vi "Launch Chart.vi"   [LabVIEW 2017]
uses:
  ExampleSimpleRootModel/SimpleRootModel.lvclass
  C:/Git/mva-framework/gpm_packages/@cs/mva-core/Source/IObserver/IObserver/IObserver.lvclass
  C:/Git/mva-framework/gpm_packages/@cs/mva-core/Source/IModel/IModel/IModel.lvclass
  SimpleChart/SimpleChart.lvclass
  C:/Git/mva-framework/gpm_packages/@cs/mva-viewable/Source/IViewable/IViewable/IViewable.lvclass
  gpm_packages/@cs/mva-viewable/Source/IViewModel/IViewModel/IViewModel.lvclass
  C:/Git/mva-framework/gpm_packages/@cs/mva-viewable/Source/IViewManager/IViewManager/IViewManager.lvclass
  C:/Program Files (x86)/National Instruments/LabVIEW 2017/vi.lib/ActorFramework/Actor/Actor.lvclass
  gpm_packages/@cs/mva-core/Source/Mediator/Mediator/Mediator.lvclass
  C:/Git/mva-framework/gpm_packages/@cs/mva-core/Source/IMediator/IMediator/IMediator.lvclass
  <vilib>/ActorFramework/Message Enqueuer/Message Priority.ctl
  gpm_packages/@cs/mva-viewable/Source/IViewable/IViewable/View Position Enum.ctl
  ExampleSimpleRootModel/SimpleRootModel.lvclass/SimpleRootModel.ctl
  gpm_packages/@cs/event-logger/Source/Composed Log/LoggerReference/LoggerReference.lvclass/LoggerReference.ctl
  gpm_packages/@cs/mva-core/Source/IObserver/IObserver/IObserver.lvclass/IObserver.ctl
  gpm_packages/@cs/mva-core/Source/IMediator/IMediator/IMediator.lvclass/IMediator.ctl
  gpm_packages/@cs/mva-viewable/Source/IViewModel/IViewModel/IViewModel.lvclass/IViewModel.ctl
  gpm_packages/@cs/mva-viewable/Source/IViewManager/IViewManager Messages/Launch Nested Views Msg/Launch Nested Views Msg.lvclass/Launch Nested Views Msg.ctl
  gpm_packages/@cs/mva-viewable/Source/IViewManager/IViewManager/IViewManager.lvclass/IViewManager.ctl
  gpm_packages/@cs/mva-viewable/Source/IViewable/IViewable Messages/Open Front Panel Msg/Open Front Panel Msg.lvclass/Open Front Panel Msg.ctl
  <vilib>/ActorFramework/Message Enqueuer/Message Enqueuer.lvclass/Message Enqueuer.ctl
  158084ce-0d1a-4c6f-81cb-d0b1039f64dd.vi
  158084ce-0d1a-4c6f-81cb-d0b1039f64dd.vi/7a735fd6-0766-4914-b472-33d23f5eb4e6.vi
  gpm_packages/@cs/mva-core/Source/IObserver/IObserver/Configure Observer Logging.vi
  gpm_packages/@cs/mva-viewable/Source/IViewModel/IViewModel/Write Startup Model-View Configuration.vi
  gpm_packages/@cs/mva-core/Source/IMediator/IMediator/Configure Mediator.vi
  <vilib>/ActorFramework/Message Enqueuer/Enqueue.vi
  gpm_packages/@cs/event-logger/Source/Composed Log/LoggerReference/Return Aggregate Queues.vi
  gpm_packages/@cs/event-logger/Source/Composed Log/LoggerReference/Add Aggregate Log.vi
  158084ce-0d1a-4c6f-81cb-d0b1039f64dd.vi/7a735fd6-0766-4914-b472-33d23f5eb4e6.vi/481b5bb9-d2a3-4a79-b1b5-84a351928f52.vi
  gpm_packages/@cs/mva-viewable/Source/IViewManager/IViewManager Messages/Launch Nested Views Msg/Pack Launch Nested Views Msg.vi
  gpm_packages/@cs/mva-viewable/Source/IViewManager/IViewManager/Write Startup Launch Nested Views Msg.vi
  gpm_packages/@cs/event-logger/Source/Composed Log/LoggerReference/Send Add Sink.vi
  gpm_packages/@cs/event-logger/Source/Text File Sink/Text File Sink.lvclass
  C:/Git/mva-framework/gpm_packages/@cs/event-logger/Source/Composed Log/Log Sink/Log Sink.lvclass
  gpm_packages/@cs/mva-viewable/Source/IViewable/IViewable Messages/Open Front Panel Msg/Open Front Panel Msg.lvclass
  C:/Program Files (x86)/National Instruments/LabVIEW 2017/vi.lib/ActorFramework/Message/Message.lvclass
  gpm_packages/@cs/event-logger/Source/Composed Log/Application Logger/Launch Worker Loop.vi
  gpm_packages/@cs/event-logger/Source/Composed Log/LoggerReference/Initialize Logger Instance.vi
  <vilib>/ActorFramework/Message Priority Queue/Priority Enqueue.vi
  gpm_packages/@cs/event-logger/Source/Composed Log/LoggerReference/LoggerReference.lvclass
  gpm_packages/@cs/event-logger/Source/Composed Log/IErrorFormat/IErrorFormat.lvclass
  gpm_packages/@cs/event-logger/Source/Composed Log/Log Sink/Log Sink.lvclass
  gpm_packages/@cs/mva-viewable/Source/IViewable/IApplicationStyle/IApplicationStyle.lvclass
  gpm_packages/@cs/mva-viewable/Source/IViewManager/IViewManager Messages/Launch Nested Views Msg/Launch Nested Views Msg.lvclass
  <vilib>/ActorFramework/Actor/Actor.lvclass
  <vilib>/ActorFramework/Message Enqueuer/Message Enqueuer.lvclass
  gpm_packages/@cs/mva-viewable/Source/IViewable/IViewable/IViewable.lvclass
panel:
  # "This example launches a simple chart MVA application"
types:
  T1 = typedef "IViewable.lvlib/IViewable.lvclass/View Position Enum.ctl" = enum16{"Centered", "Maximized", "Minimized", "Custom", "Unchanged"}
  T2 = typedef "Actor Framework.lvlib/Message Enqueuer.lvclass/Message Priority.ctl" = enum16{"Low", "Normal", "High"}
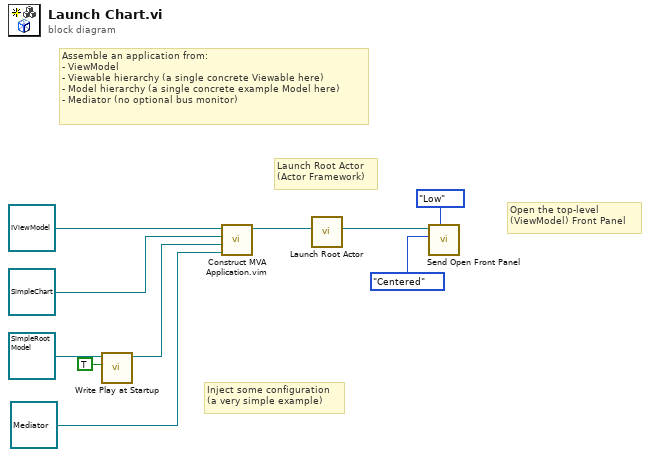
[diagram p0: block diagram]
diagram:
  # "Inject some configuration\n(a very simple example)"
  # "Open the top-level\n(ViewModel) Front Panel"
  # "Launch Root Actor\n(Actor Framework)"
  # "Assemble an application from:\n- ViewModel\n- Viewable hierarchy (a single concrete Viewable here)\n- Model hierarchy (a single concrete example Model here)\n- Mediator (no optional bus monitor)"
  n1 = call "Write Play at Startup.vi"("Play at Startup?"=TRUE, "SimpleRootModel in"=refnum<class "SimpleRootModel.lvclass"> refnum ("MVAExamples.lvlib:SimpleRootModel.lvclass")) -> ("SimpleRootModel out"=w3:refnum<class "SimpleRootModel.lvclass">)  [unwired: 9 in]
  n2 = call "Construct MVA Application.vim"("Mediator Type"=refnum<class "Mediator.lvclass"> refnum ("Mediator.lvlib:Mediator.lvclass"), "Model Type"=w3, "Startup View Configuration"=refnum<class "SimpleChart.lvclass"> refnum ("MVAExamples.lvlib:SimpleChart.lvclass"), "IViewModel In"=refnum<class "IViewModel.lvclass"> refnum ("IViewModel.lvlib:IViewModel.lvclass")) -> ("IViewModel Out"=w7:refnum<class "IViewModel.lvclass">)  [unwired: 7 in]
  n3 = call <vilib>:"Launch Root Actor.vi"("Actor"=w7) -> ("Actor's Enqueuer"=w6:refnum<class "Message Enqueuer.lvclass">)  [unwired: 9 in, 1 out]
  n4 = call "Send Open Front Panel.vi"("Message Priority (Normal)"=Message_Priority."Low", "Position"=View_Position_Enum."Centered", "Message Enqueuer"=w6) -> ()  [unwired: 7 in, 2 out]
